vi "solar_misc Unpack LLB.vi"() -> ()   [LabVIEW 2018]
doc: "This unpacks an LLB into individual files."
panel:
  in  "LLB Path (*.llb)":path=path "C:/Data/agn6700.llb"
  out "All Files in Dir":path[](array[path])
  out "error out":errorcluster
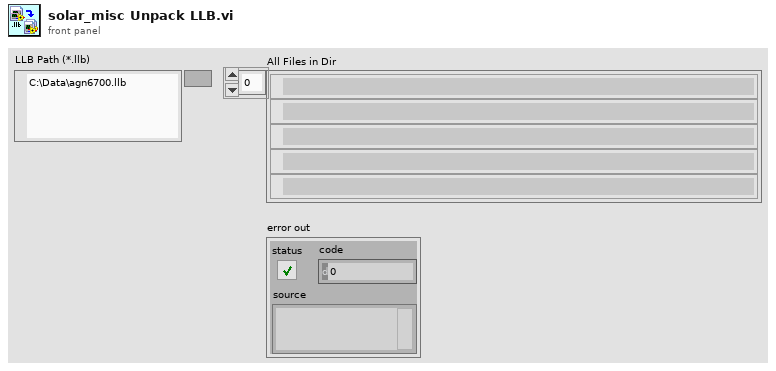
[diagram p1: front panel]
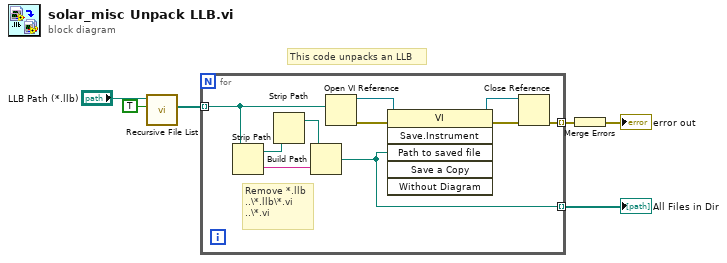
[diagram p0: block diagram]
diagram:
  # "This code unpacks an LLB"
  n1 = call <vilib>:"Recursive File List.vi"("Treat LLBs as Folders?"=TRUE, "Folder Path"="LLB Path (*.llb)") -> ("All Files in Dir"=w4:path[])  [unwired: 5 in, 4 out]
  n2 = for {
    tunnel: w4 -> [w14] mode=indexing
    tunnel: [w8] -> w3 mode=indexing
    tunnel: [w7] -> w2 mode=indexing
    # "Remove *.llb\n..\\*.llb\\*.vi\n..\\*.vi"
    n3 = Strip Path(path=w14) -> (stripped path=w13:path, name=w11:string)
    n4 = Strip Path(path=w13) -> (stripped path=w12:path)  [unwired: 1 out]
    n5 = Build Path(base path=w12, name or relative path=w11) -> (appended path=w7:path)
    n6 = Open VI Reference(vi path=w14) -> (vi reference=w15:refnum<vi>, error out=w16:errorcluster)  [unwired: 5 in]
    n7 = invoke class="VI" method="Save.Instrument"(reference=w15, error in=w16, "Path to saved file"=w7) -> (reference out=w9:refnum<vi>, error out=w10:errorcluster)  [unwired: 3 in, 4 out]
    n8 = Close Reference(reference=w9, error in (no error)=w10) -> (error out=w8:errorcluster)
  }
  "All Files in Dir" <- w2
  n9 = Merge Errors(w3) -> (→"error out":errorcluster)
